vi "Find Intensity Peaks V3.vi"(4 "Gaussian Fit Method":T2 items=["Least Square", "Least Absolute Residual", "Bisquare"], 5 "Padding":u32=3, 6 "error in (no error)":errorcluster, 7 "Target Baseline (%)":dbl=10.0, 8 "Intensity Threshold":i32, 9 "Data In":dbl[](array[numeric])) -> (0 "error out":errorcluster, 1 "Valid Fit?":bool, 2 "Gaussian Fit Parameters":T1, 3 "All Data (X,Y)":cluster{"Locations":dbl[], "Amplitudes":dbl[]}[](array[cluster]))   [LabVIEW 2012]
doc: "Algorithm doesn't handle clipped pulses"
uses:
  <vilib>/Analysis/6fits.llb/Curve Fitting Criteria.ctl
  <vilib>/Analysis/NI_AAL_SigProc.lvlib
  <vilib>/Analysis/NI_AALPro.lvlib
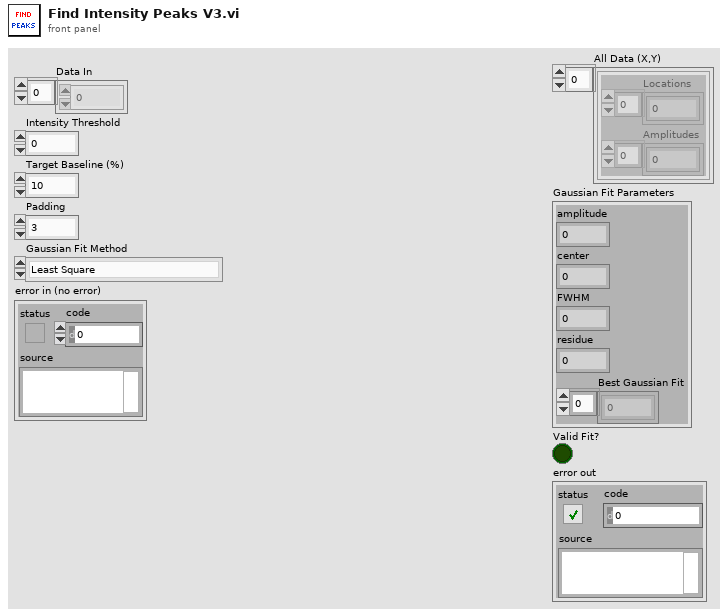
[diagram p1: front panel]
types:
  T1 = cluster{"amplitude":dbl, "center":dbl, "FWHM":dbl, "residue":dbl, "Best Gaussian Fit":dbl[]}
  T2 = typedef "NI_AALPro.lvlib/Curve Fitting Criteria.ctl" = u16
  T3 = cluster{"Indices":u32[], "Best Gaussian Fit":dbl[]}
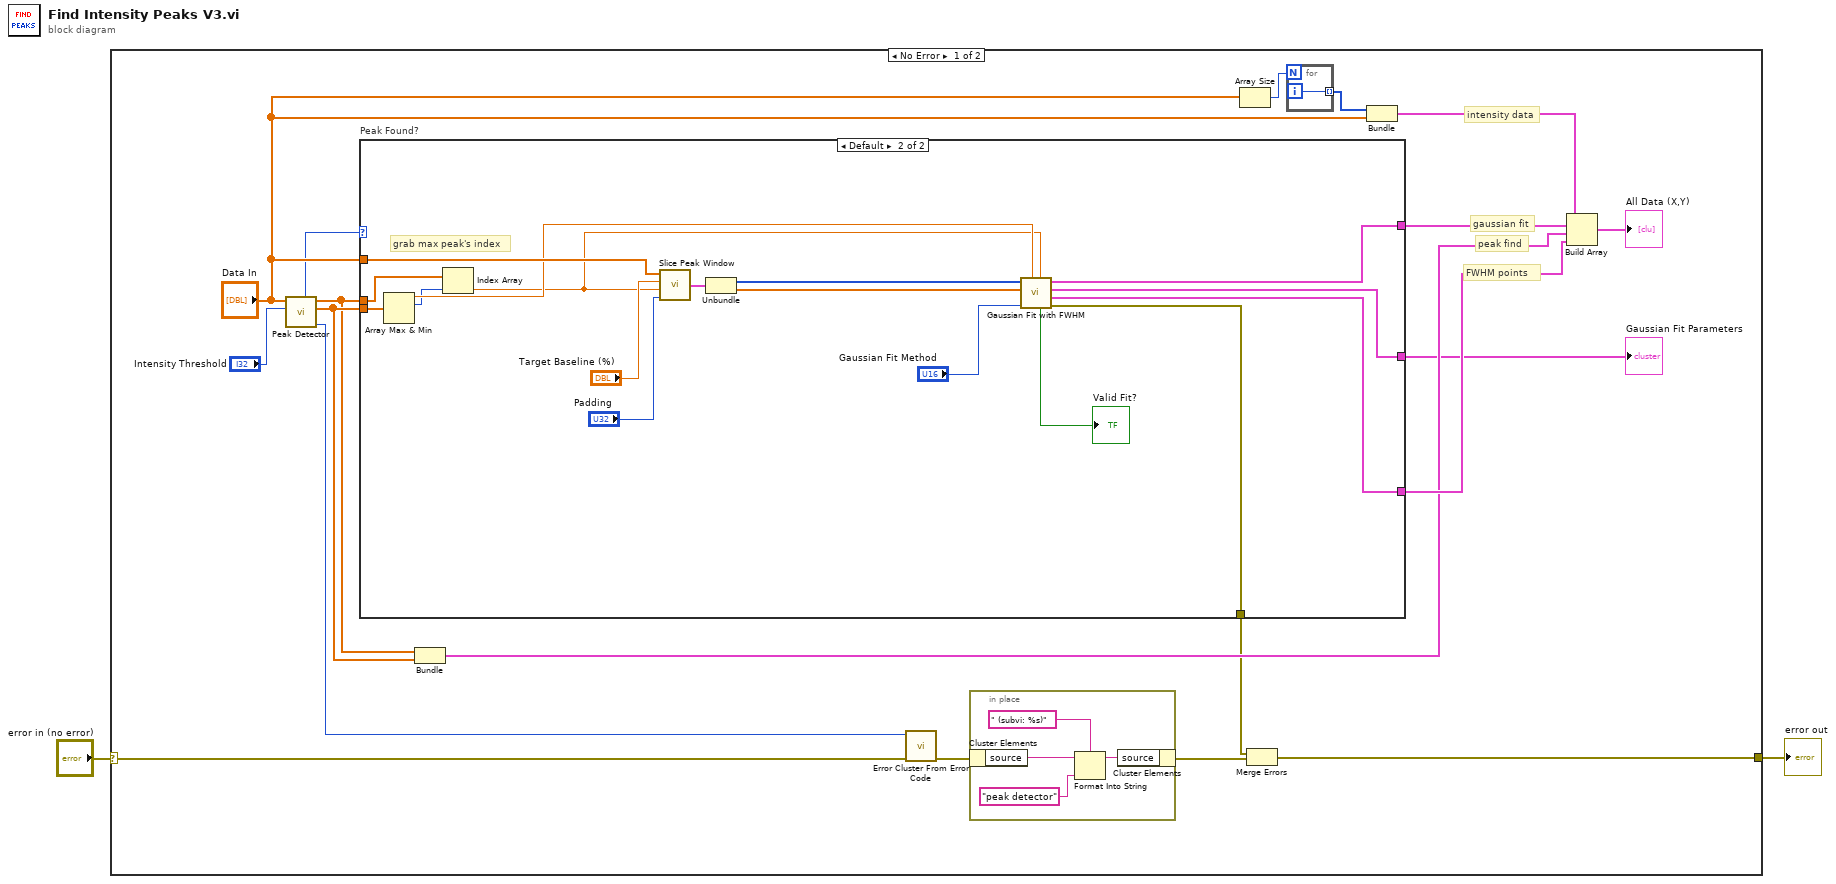
[diagram p0: block diagram]
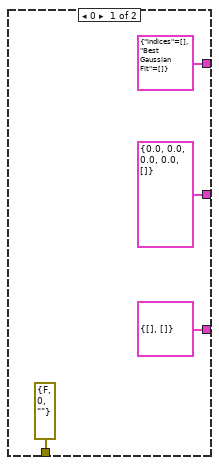
[diagram p2: hidden frame]
diagram:
  n1 = case shown="No Error" "error in (no error)" {
    selector: "error in (no error)" -> [w10 w48]
    tunnel: [w11 w48] -> w2
    frame No Error {
      # "FWHM points"
      # "peak find"
      # "gaussian fit"
      # "intensity data"
      n2 = call <vilib>:"Peak Detector.vi"("threshold"="Intensity Threshold", "X"="Data In") -> ("error"=w17:i32, "Amplitudes"=w8:dbl[], "Locations"=w7:dbl[], "# found"=w5:i32)  [unwired: 5 in, 1 out]
      n3 = case "Peak Found?" shown="Default" w5 {
        tunnel: [T3 {"Indices"=[], "Best Gaussian Fit"=[]} w42] -> w19
        tunnel: [cluster{dbl[], dbl[]} {[], []} w41] -> w14
        tunnel: "Data In" -> [_ w40]
        tunnel: w8 -> [_ w34]
        tunnel: w7 -> [_ w33]
        tunnel: [T1 {"amplitude"=0.0, "center"=0.0, "FWHM"=0.0, "residue"=0.0, "Best Gaussian Fit"=[]} ("Gaussian Fit Data") w31] -> w4
        tunnel: [errorcluster {"status"=FALSE, "code"=0, "source"=""} ("error out") w30] -> w3
        frame 0 {
        }
        frame Default {
          # "grab max peak's index"
          n4 = Array Max & Min(array=w34) -> (max value=w35:dbl, max index (indices)=w28:i32)  [unwired: 2 out]
          n5 = Index Array(array=w33, index=w28) -> (element=w27:dbl)
          n6 = call "Slice Peak Window.vi"("Padding"="Padding", "Peak Index"=w27, "Target Baseline (%)"="Target Baseline (%)", "Intensity Data"=w40) -> ("Peak Window (X,Y)"=w37:cluster{"Indices":u32[], "Sliced Data":dbl[]})
          n7 = Unbundle(w37) -> ("Indices"=w32:u32[], "Sliced Data"=w36:dbl[])
          n8 = call "Gaussian Fit with FWHM.vi"("Initial Center"=w27, "Inital Amplitude"=w35, "Gaussian Fit Method"="Gaussian Fit Method", "Y data"=w36, "X data"=w32) -> ("error out"=w30:errorcluster, "FWHM (X,Y)"=w41:cluster{dbl[], dbl[]}, "Gaussian Fit Data"=w31:T1, "Gaussian Fit (X,Y)"=w42:T3, "Valid Fit?"=→"Valid Fit?":bool)  [unwired: 2 in]
        }
      }
      "Gaussian Fit Parameters" <- w4
      n9 = Bundle("Locations"=w7, "Amplitudes"=w8) -> (w6:cluster{"Locations":dbl[], "Amplitudes":dbl[]})  [unwired: 1 in]
      n10 = call <vilib>:"Error Cluster From Error Code.vi"("error in (no error)"=w10, "error code (0)"=w17) -> ("error out"=w13:errorcluster)  [unwired: 7 in]
      n11 = in-place "In Place Element Structure" {
        n12 = in-place-cluster #1(w13) -> ("source"=w44:string)
        n13 = Format Into String(format string=" (subvi: %s)" ("initial string"), initial string=w44, "peak detector" ("input 1")) -> (resulting string=w46:string)  [unwired: 1 in, 1 out]
        n14 = in-place-cluster #1("source"=w46) -> (w12:errorcluster)
      }
      n15 = Array Size(array="Data In") -> (size(s)=w16:i32)
      n16 = Merge Errors(w3, w12) -> (w11:errorcluster)
      n17 = for {
        N: w16 -> [_]
        tunnel: [w47] -> w15 mode=indexing
        i -> [w47]
      }
      n18 = Bundle(w15, "Data In"="Data In") -> (w18:cluster{i32[], "Data In":dbl[]})  [unwired: 1 in]
      n19 = Build Array(w18, w19, w6, w14) -> (→"All Data (X,Y)":cluster{"Locations":dbl[], "Amplitudes":dbl[]}[])
    }
    frame Error {
    }
  }
  "error out" <- w2
